vi "Registry.vi"(7 "action":T1, 11 "data in":variant) -> (0 "error out":errorcluster, 3 "data out":variant)   [LabVIEW 2024, in "Logging.lvlib" / "Registry.lvlib"]
uses:
  Registry.lvlib
  Registry Actions.ctl
  Logger/Logger.lvclass
  Logger/Logger.lvclass/Logger.ctl
  Log Action Data.ctl
  Log Levels.ctl
  <vilib>/Utility/error.llb/Error Cluster From Error Code.vi
  <vilib>/ErrorRing/Error Ring.xnode
  Logging.lvlib
  Utilities/Utilities.lvlib
panel:
  # "Connector Pane"
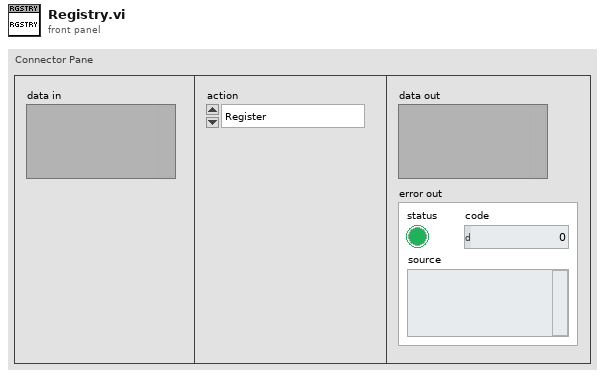
[diagram p1: front panel]
types:
  T1 = typedef "Logging.lvlib/Registry.lvlib/Registry Actions.ctl" = enum16{"Register", "Log", "Enable", "Enable All", "Disable", "Disable All", "List", "Unregister", "Unregister All"}
  T2 = typedef "Logging.lvlib/Registry.lvlib/Log Action Data.ctl" = cluster{"level":T3, "message":string, "data":variant}
  T3 = typedef "Logging.lvlib/Log Levels.ctl" = enum16{"Trace", "Debug", "Info", "Warning", "Error", "Critical"}
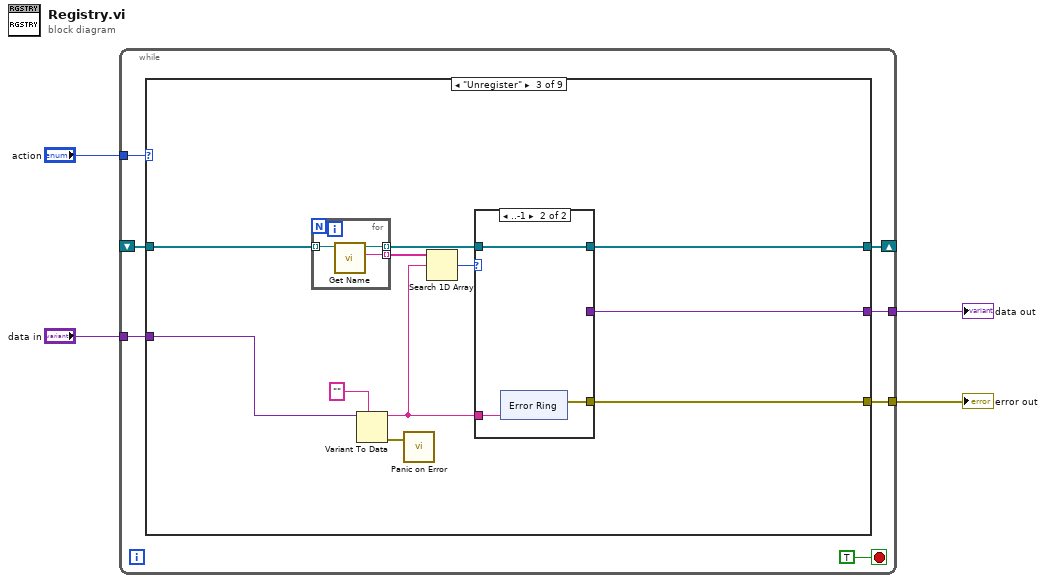
[diagram p0: block diagram]
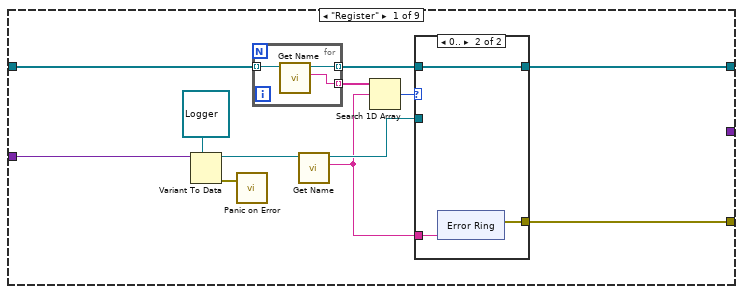
[diagram p2: hidden frame]
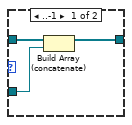
[diagram p3: hidden frame]
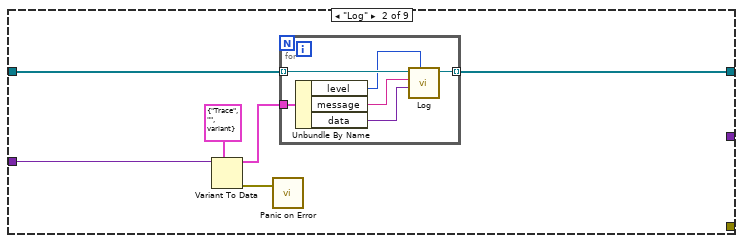
[diagram p4: hidden frame]
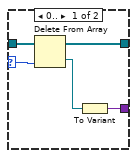
[diagram p5: hidden frame]
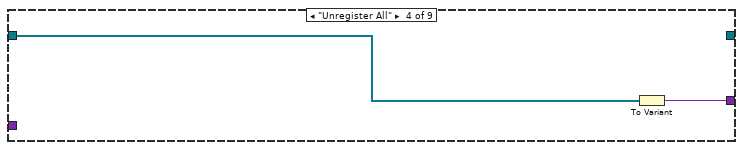
[diagram p6: hidden frame]
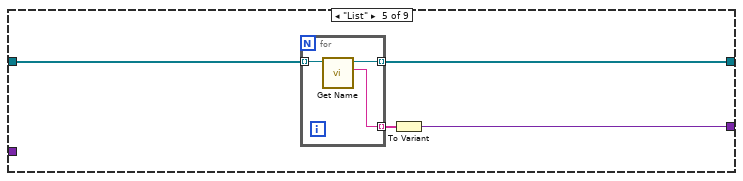
[diagram p7: hidden frame]
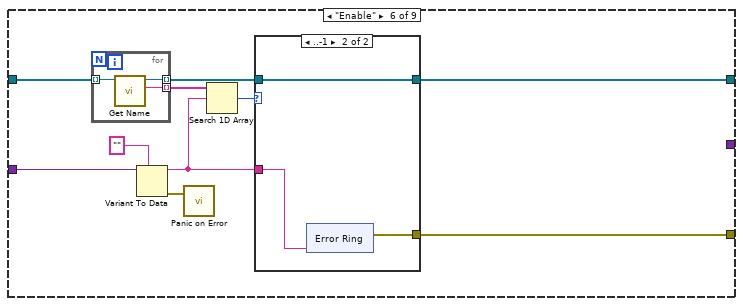
[diagram p8: hidden frame]
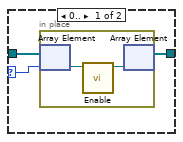
[diagram p9: hidden frame]
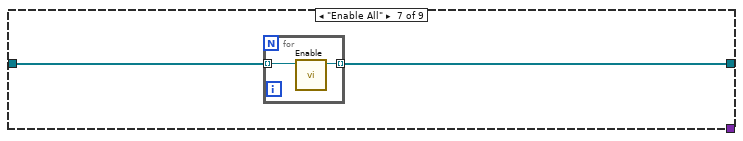
[diagram p10: hidden frame]
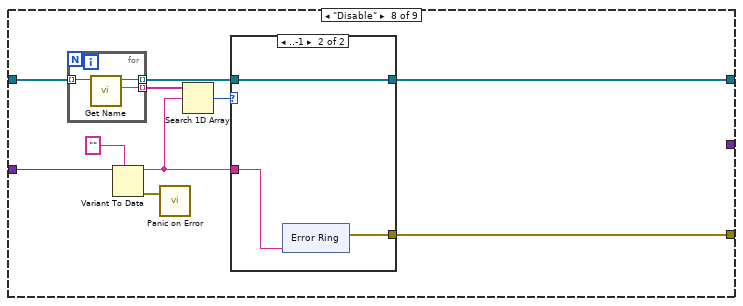
[diagram p11: hidden frame]
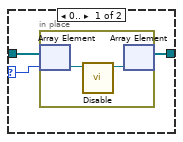
[diagram p12: hidden frame]
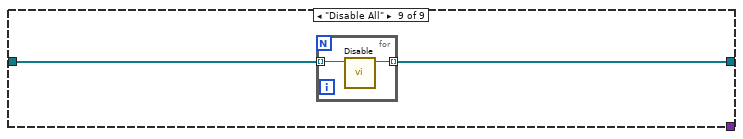
[diagram p13: hidden frame]
diagram:
  n1 = while {
    tunnel: "action" -> [w10]
    tunnel: "data in" -> [w9]
    shift-right: [w8] -> _
    shift-left: _ -> [w7]
    tunnel: [w6] -> w2
    tunnel: [w5] -> w1
    stop <- TRUE stop-if-true
    n2 = case shown="\"Unregister\"" w10 {
      tunnel: w9 -> [w23 w44 w61 _ _ w90 _ w124 _]
      tunnel: [w21 w41 w56 _ w85 w92 w118 w123 w150] -> w8
      tunnel: w7 -> [w19 w45 w62 w82 w86 w93 w119 w125 w151]
      tunnel: [_ _ w55 w81 w83 _ _ _ _] -> w6
      tunnel: [w13 _ w53 _ _ w91 _ w122 _] -> w5
      frame "Register" {
        n3 = Variant To Data(type=refnum<class "Logger.lvclass"> refnum ("Logging.lvlib:Logger.lvclass"), Variant=w23) -> (data=w17:refnum<class "Logger.lvclass">, error out=w12:errorcluster)  [unwired: 1 in]
        n4 = call "Panic on Error.vi"("error in (no error)"=w12) -> ()  [unwired: 3 in]
        n5 = for {
          tunnel: w19 -> [w39] mode=indexing
          tunnel: [w38] -> w20 mode=indexing
          tunnel: [w37] -> w18 mode=indexing
          n6 = call "Get Name.vi"("logger in"=w39) -> ("name"=w37:string, "logger out"=w38:refnum<class "Logger.lvclass">)  [unwired: 9 in]
        }
        n7 = call "Get Name.vi"("logger in"=w17) -> ("name"=w14:string, "logger out"=w16:refnum<class "Logger.lvclass">)  [unwired: 9 in]
        n8 = Search 1D Array(1D array=w18, element=w14) -> (index of element=w15:i32)  [unwired: 1 in]
        n9 = case shown="0.." w15 {
          tunnel: [w26 w29] -> w21
          tunnel: w20 -> [w25 w29]
          tunnel: w16 -> [w24 _]
          tunnel: w14 -> [_ w28]
          tunnel: [_ w27] -> w13
          frame ..-1 {
            n10 = Build Array (concatenate)(w25, w24) -> (w26:refnum<class "Logger.lvclass">[])
          }
          frame 0.. {
            n11 = xnode "Error Ring"("parameter 0"=w28) -> ("error out"=w27:errorcluster)
          }
        }
      }
      frame "Log" {
        n12 = Variant To Data(type=T2 {"level"=enum."Trace", "message"="", "data"=variant}, Variant=w44) -> (data=w42:T2, error out=w40:errorcluster)  [unwired: 1 in]
        n13 = call "Panic on Error.vi"("error in (no error)"=w40) -> ()  [unwired: 3 in]
        n14 = for {
          tunnel: w45 -> [w51] mode=indexing
          tunnel: w42 -> [w50]
          tunnel: [w46] -> w41 mode=indexing
          n15 = Unbundle By Name(w50) -> ("level"=w49:T3, "message"=w48:string, "data"=w47:variant)
          n16 = call "Log.vi"("log level"=w49, "data (null)"=w47, "message"=w48, "logger in"=w51) -> ("logger out"=w46:refnum<class "Logger.lvclass">)  [unwired: 7 in]
        }
      }
      frame "Unregister" {
        n17 = for {
          tunnel: w62 -> [w80] mode=indexing
          tunnel: [w79] -> w59 mode=indexing
          tunnel: [w78] -> w57 mode=indexing
          n18 = call "Get Name.vi"("logger in"=w80) -> ("name"=w79:string, "logger out"=w78:refnum<class "Logger.lvclass">)  [unwired: 9 in]
        }
        n19 = Variant To Data(type="", Variant=w61) -> (data=w54:string, error out=w52:errorcluster)  [unwired: 1 in]
        n20 = call "Panic on Error.vi"("error in (no error)"=w52) -> ()  [unwired: 3 in]
        n21 = Search 1D Array(1D array=w59, element=w54) -> (index of element=w58:i32)  [unwired: 1 in]
        n22 = case shown="..-1" w58 {
          selector: w58 -> [w66 _]
          tunnel: w57 -> [w67 w70]
          tunnel: [w65 w70] -> w56
          tunnel: [w63 _] -> w55
          tunnel: w54 -> [_ w69]
          tunnel: [_ w68] -> w53
          frame 0.. {
            n23 = Delete From Array(array=w67, index=w66) -> (deleted portion=w64:refnum<class "Logger.lvclass">, array with subset deleted=w65:refnum<class "Logger.lvclass">[])  [unwired: 1 in]
            n24 = To Variant(anything=w64) -> (Variant=w63:variant)
          }
          frame ..-1 {
            n25 = xnode "Error Ring"("parameter 0"=w69) -> ("error out"=w68:errorcluster)
          }
        }
      }
      frame "Unregister All" {
        n26 = To Variant(anything=w82) -> (Variant=w81:variant)
      }
      frame "List" {
        n27 = for {
          tunnel: w86 -> [w89] mode=indexing
          tunnel: [w88] -> w85 mode=indexing
          tunnel: [w87] -> w84 mode=indexing
          n28 = call "Get Name.vi"("logger in"=w89) -> ("name"=w87:string, "logger out"=w88:refnum<class "Logger.lvclass">)  [unwired: 9 in]
        }
        n29 = To Variant(anything=w84) -> (Variant=w83:variant)
      }
      frame "Enable" {
        n30 = for {
          tunnel: w93 -> [w117] mode=indexing
          tunnel: [w116] -> w98 mode=indexing
          tunnel: [w115] -> w96 mode=indexing
          n31 = call "Get Name.vi"("logger in"=w117) -> ("name"=w116:string, "logger out"=w115:refnum<class "Logger.lvclass">)  [unwired: 9 in]
        }
        n32 = Variant To Data(type="", Variant=w90) -> (data=w95:string, error out=w94:errorcluster)  [unwired: 1 in]
        n33 = call "Panic on Error.vi"("error in (no error)"=w94) -> ()  [unwired: 3 in]
        n34 = Search 1D Array(1D array=w98, element=w95) -> (index of element=w97:i32)  [unwired: 1 in]
        n35 = case shown="..-1" w97 {
          selector: w97 -> [w101 _]
          tunnel: w96 -> [w102 w107]
          tunnel: [w100 w107] -> w92
          tunnel: w95 -> [_ w106]
          tunnel: [_ w105] -> w91
          frame 0.. {
            n36 = in-place {
              n37 = in-place-array #1(w102, w101) -> (w104:refnum<class "Logger.lvclass">)
              n38 = call "Enable.vi"("logger in"=w104) -> ("logger out"=w103:refnum<class "Logger.lvclass">)  [unwired: 10 in]
              n39 = in-place-array #1(w103) -> (w100:refnum<class "Logger.lvclass">[])  [unwired: 1 out]
            }
          }
          frame ..-1 {
            n40 = xnode "Error Ring"("parameter 0"=w106) -> ("error out"=w105:errorcluster)
          }
        }
      }
      frame "Enable All" {
        n41 = for {
          tunnel: w119 -> [w121] mode=indexing
          tunnel: [w120] -> w118 mode=indexing
          n42 = call "Enable.vi"("logger in"=w121) -> ("logger out"=w120:refnum<class "Logger.lvclass">)  [unwired: 10 in]
        }
      }
      frame "Disable" {
        n43 = for {
          tunnel: w125 -> [w149] mode=indexing
          tunnel: [w148] -> w130 mode=indexing
          tunnel: [w147] -> w128 mode=indexing
          n44 = call "Get Name.vi"("logger in"=w149) -> ("name"=w148:string, "logger out"=w147:refnum<class "Logger.lvclass">)  [unwired: 9 in]
        }
        n45 = Variant To Data(type="", Variant=w124) -> (data=w127:string, error out=w126:errorcluster)  [unwired: 1 in]
        n46 = call "Panic on Error.vi"("error in (no error)"=w126) -> ()  [unwired: 3 in]
        n47 = Search 1D Array(1D array=w130, element=w127) -> (index of element=w129:i32)  [unwired: 1 in]
        n48 = case shown="..-1" w129 {
          selector: w129 -> [w133 _]
          tunnel: w128 -> [w134 w139]
          tunnel: [w132 w139] -> w123
          tunnel: w127 -> [_ w138]
          tunnel: [_ w137] -> w122
          frame 0.. {
            n49 = in-place {
              n50 = in-place-array #2(w134, w133) -> (w136:refnum<class "Logger.lvclass">)
              n51 = call "Disable.vi"("logger in"=w136) -> ("logger out"=w135:refnum<class "Logger.lvclass">)  [unwired: 10 in]
              n52 = in-place-array #2(w135) -> (w132:refnum<class "Logger.lvclass">[])  [unwired: 1 out]
            }
          }
          frame ..-1 {
            n53 = xnode "Error Ring"("parameter 0"=w138) -> ("error out"=w137:errorcluster)
          }
        }
      }
      frame "Disable All" {
        n54 = for {
          tunnel: w151 -> [w153] mode=indexing
          tunnel: [w152] -> w150 mode=indexing
          n55 = call "Disable.vi"("logger in"=w153) -> ("logger out"=w152:refnum<class "Logger.lvclass">)  [unwired: 10 in]
        }
      }
    }
  }
  "data out" <- w2
  "error out" <- w1
